vi "Cheesy Drive.vi"(2 "Quick Turn":bool, 3 "Turn":dbl, 4 "Throttle":dbl) -> (0 "Right Motor":dbl, 1 "Left Motor":dbl)   [LabVIEW 2015]
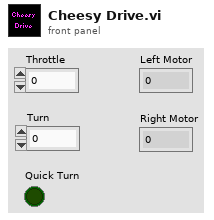
[diagram p1: front panel]
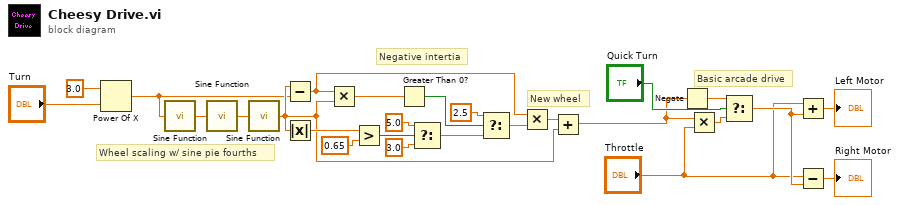
[diagram p0: block diagram]
diagram:
  # "Basic arcade drive"
  # "New wheel"
  # "Negative intertia"
  # "Wheel scaling w/ sine pie fourths"
  n1 = Power Of X(1:"Turn", 2:3.0 ("y")) -> (0:w8:dbl)
  n2 = call "Sine Function.vi"("Input"=w8) -> ("Output"=w24:dbl)
  n3 = call "Sine Function.vi"("Input"=w24) -> ("Output"=w23:dbl)
  n4 = call "Sine Function.vi"("Input"=w23) -> ("Output"=w10:dbl)
  n5 = Subtract(x=w10, y=w8) -> (x-y=w13:dbl)
  n6 = Absolute Value(x=w10) -> (abs(x)=w18:dbl)
  n7 = Multiply(x=w13, y=w10) -> (x*y=w22:dbl)
  n8 = Greater?(x=w18, y=0.65) -> (0:w19:bool)
  n9 = Greater Than 0?(x=w22) -> (x > 0?=w21:bool)
  n10 = Select(t=5.0, s=w19, f=3.0) -> (s? t:f=w14:dbl)
  n11 = Select(t=2.5, s=w21, f=w14) -> (s? t:f=w12:dbl)
  n12 = Multiply(x=w13, y=w12) -> (x*y=w11:dbl)
  n13 = Add(x=w11, y=w10) -> (x+y=w3:dbl)
  n14 = Negate(x=w3) -> (-x=w1:dbl)
  n15 = Multiply(x=w3, y="Throttle") -> (x*y=w6:dbl)
  n16 = Select(t=w1, s="Quick Turn", f=w6) -> (s? t:f=w4:dbl)
  n17 = Add(x="Throttle", y=w4) -> (x+y=→"Left Motor":dbl)
  n18 = Subtract(x="Throttle", y=w4) -> (x-y=→"Right Motor":dbl)
